vi "TDC_getTimebase.vi"() -> (3 "Time Base [s]":dbl)   [LabVIEW 2013]
uses:
  QUTAU-15_06_25/userlib/lib/tdcbase.dll
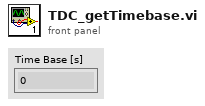
[diagram p1: front panel]
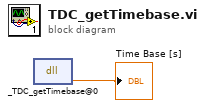
[diagram p0: block diagram]
diagram:
  n1 = dll-call lib="C:/Users/science/Desktop/NVExperimeent/Labview/QUTAU-15_06_25/userlib/lib/tdcbase.dll" fn="_TDC_getTimebase@0"() -> ("return type"=→"Time Base [s]":dbl)  [unwired: 3 in, 2 out]
